vi "FL_Preprocess_and_save_incrementally_TDMS.vi"(0 "Temporary file output path":path, 1 "Loop iteration":i32, 2 "Mouse face dir. swap":bool, 3 "Loop speed in ms":u16, 4 "Save every N seconds":u32=15, 5 "error in (no error)":errorcluster, 6 "Filter type":u16(ring)=5 items=["None", "Kalman 0.50", "Kalman 0.30", "Kalman 0.12", "Savitzky-Golay 3/5", "Savitzky-Golay 3/11", "Savitzky-Golay 3/31"], 7 "Sensor read input":T3(array[cluster]), 8 "Offset":sgl, 9 "tdms file in":refnum<k34>, 10 "Pixels per mm":dbl, 11 "Data flow controls in":T2, 12 "Diagram at recording bounds":T1, 13 "Sensor board size":string="Small") -> (14 "Eff. save interval":sgl, 15 "Latest sensor output (decoded)":string[][](array[string]), 16 "Fire TTL":bool, 17 "TTL out N":u8, 18 "Current TTL status":u8, 19 "error out":errorcluster)   [LabVIEW 2016]
uses:
  <vilib>/Utility/miscctls.llb/LVBoundsTypeDef.ctl
  SW_Globals.vi
  <vilib>/Utility/file.llb/Write Delimited Spreadsheet (string).vi
panel:
  out "Bytes return count":u32
  out "VISA error out":errorcluster
  out "Output to the external terminal":string
  in  "Max chunk size":i64=100000
  in  "Number of the file chunk":u32
  out "Chunk size (in bytes)":i64
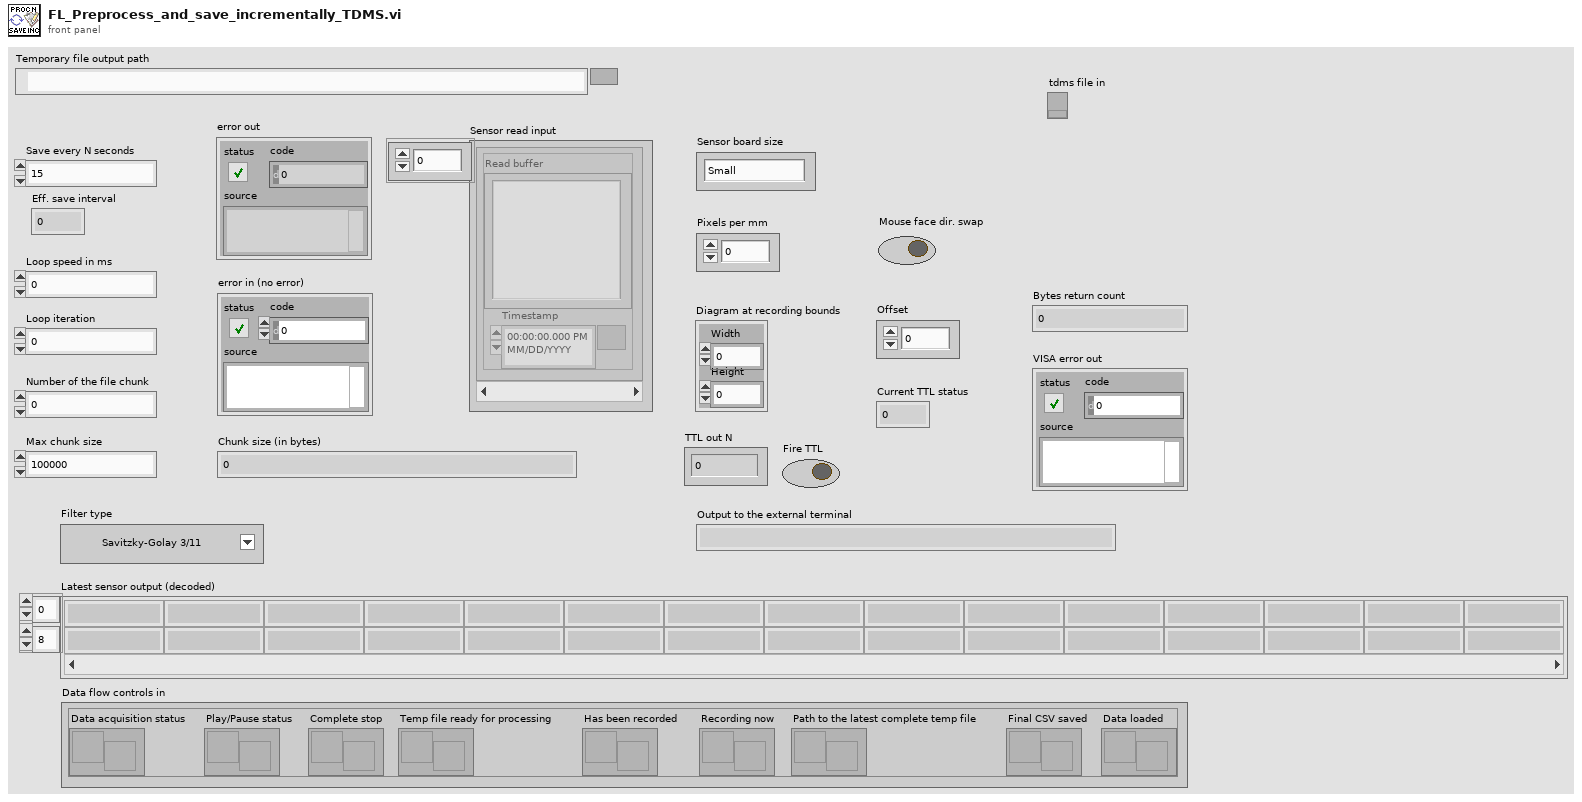
[diagram p1: front panel]
types:
  T1 = typedef "LVBoundsTypeDef.ctl" = cluster{"Width":u32, "Height":u32}
  T2 = cluster{"Data acquisition status":refnum<notifier>, "Play/Pause status":refnum<notifier>, "Complete stop":refnum<notifier>, "Temp file ready for processing":refnum<notifier>, "Has been recorded":refnum<notifier>, "Recording now":refnum<notifier>, "Path to the latest complete temp file":refnum<notifier>, "Final CSV saved":refnum<notifier>, "Data loaded":refnum<notifier>}
  T3 = cluster{"Read buffer":string, "Timestamp":timestamp}[]
  T4 = cluster{"ms since ON":u32, "delta time":u32, "X1":sgl, "Y1":sgl, "X2":sgl, "Y2":sgl, "TTL inputs":u8, "TTL outputs":u8, "Frame timestamp":timestamp, "Frame OK":bool}
  T5 = cluster{"X1 filtered":dbl, "Y1 filtered":dbl, "X2 filtered":dbl, "Y2 filtered":dbl, "X1 raw":dbl, "Y1 raw":dbl, "X2 raw":dbl, "Y2 raw":dbl}
  T6 = cluster{"R from center":dbl, "sin(a)":dbl, "Mouse Xc":dbl, "Mouse Yc":dbl, "X1-X2":dbl, "Y1-Y2":dbl, "Cage Xc":dbl, "Cage Yc":dbl}
  T7 = cluster{"R from center":dbl, "phi (mouse angular position in the cage)":dbl, "alpha (mouse rot. angle)":sgl, "X":dbl, "Y":dbl, "theta (from center towards mouse)":dbl, "beta (cage rot. against mouse)":sgl, "w (mouse angle to wall)":dbl}
  T8 = cluster{"Zone[1]":bool, "Zone[2]":bool, "Zone[3]":bool, "Zone[4]":bool, "Zone[5]":bool, "Zone[6]":bool, "Zone[7]":bool, "Zone[8]":bool, "Zone[9]":bool, "Zone[10]":bool, "Zone[11]":bool, "Zone[12]":bool, "Zone[13]":bool}
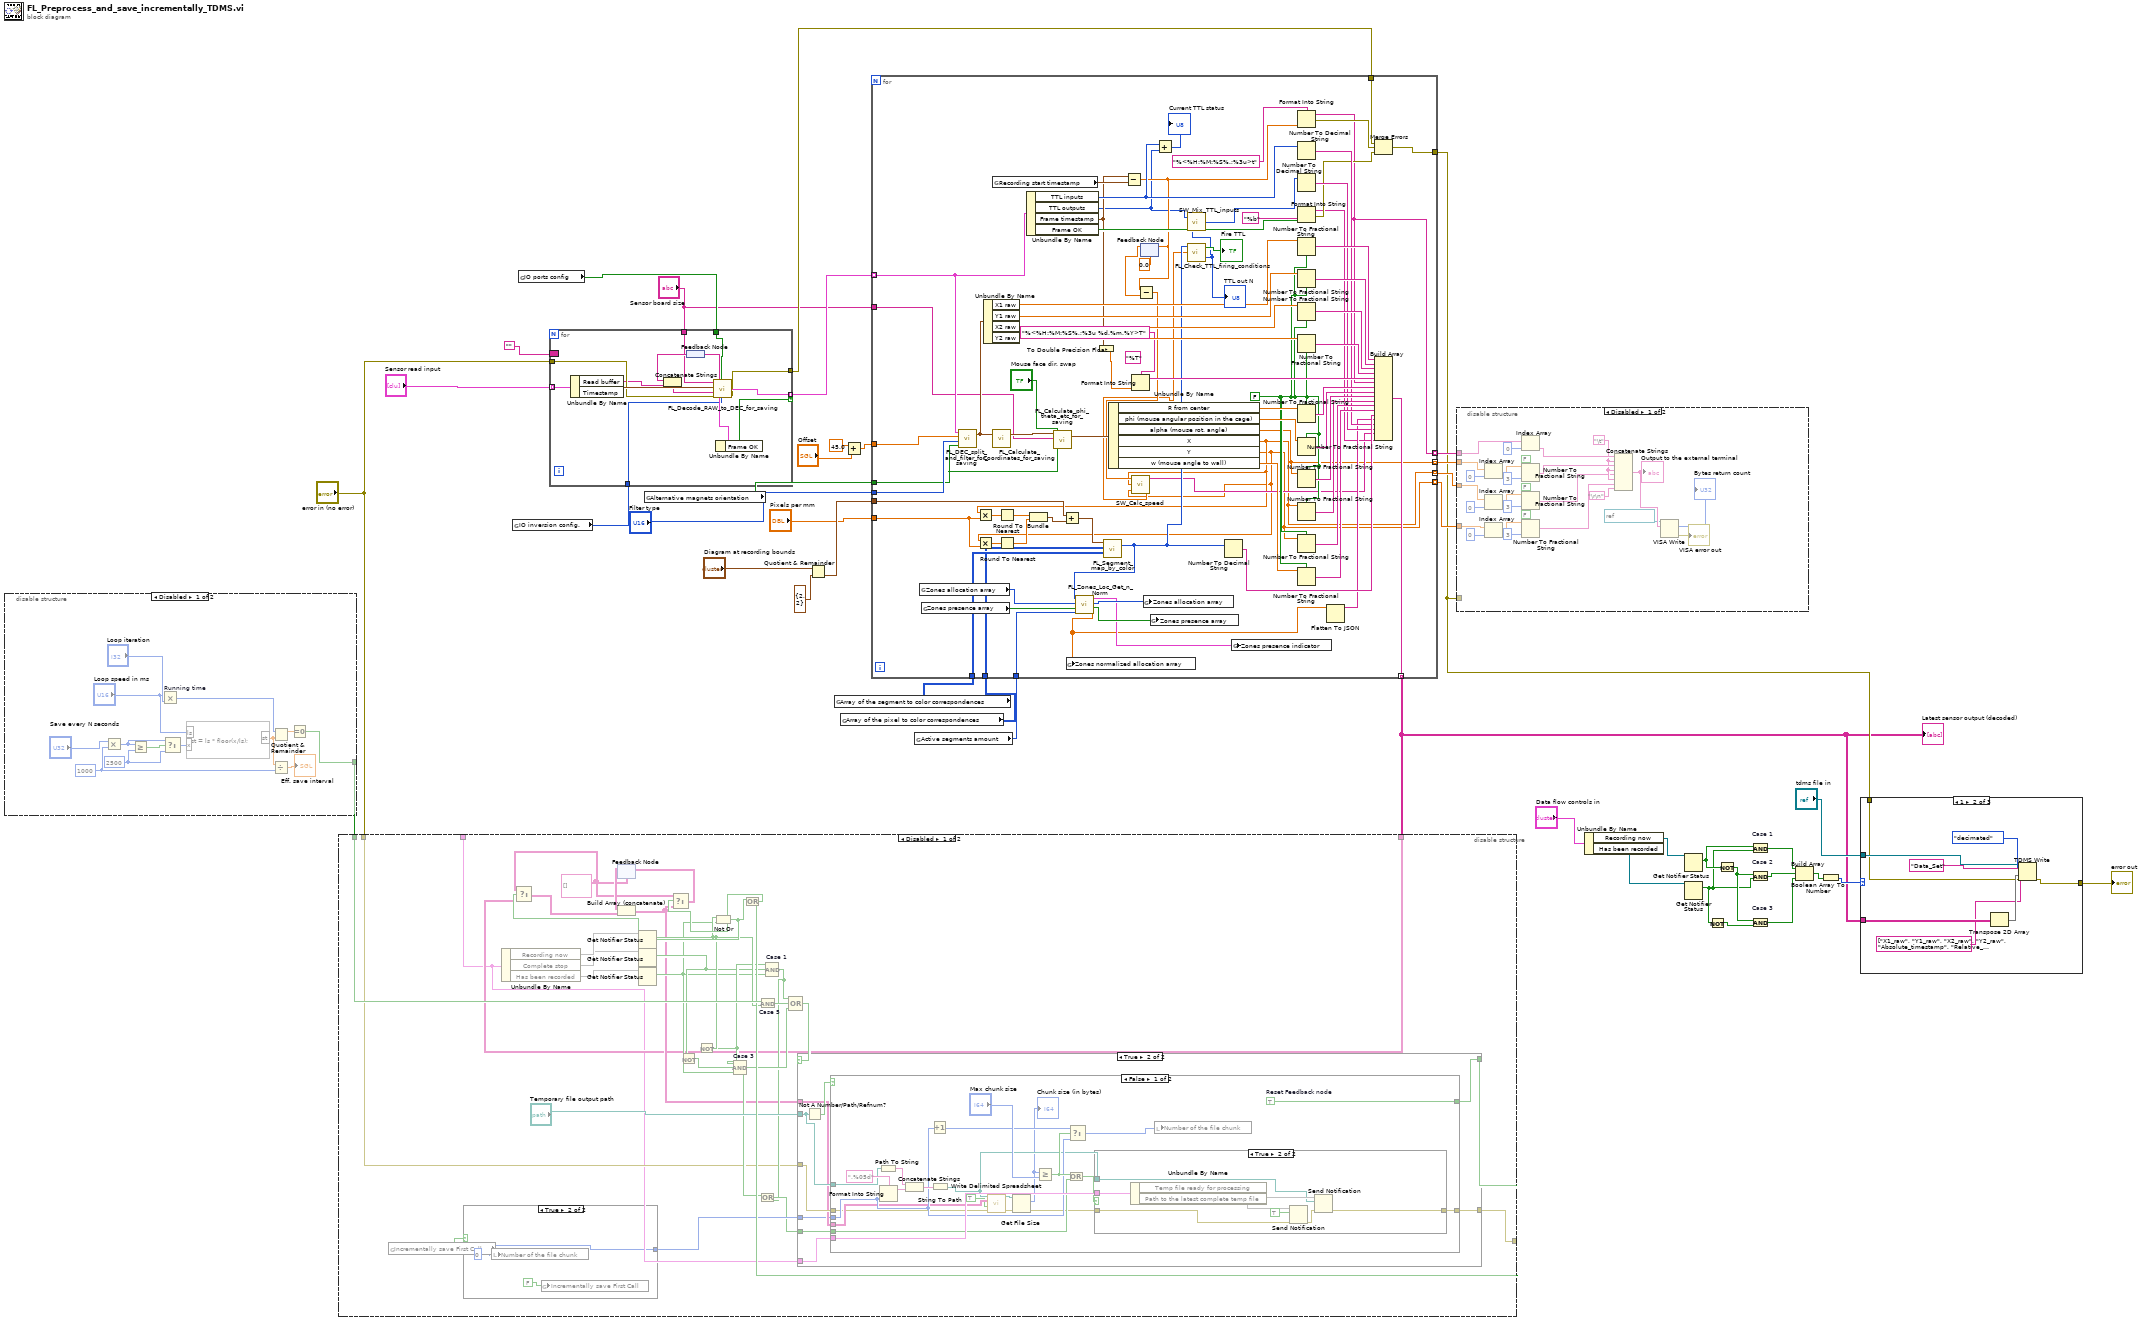
[diagram p0: block diagram]
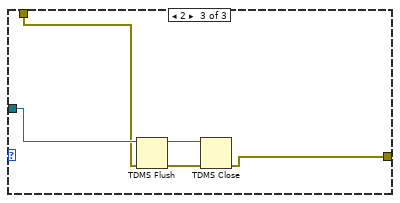
[diagram p3: hidden frame]
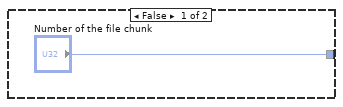
[diagram p4: hidden frame]
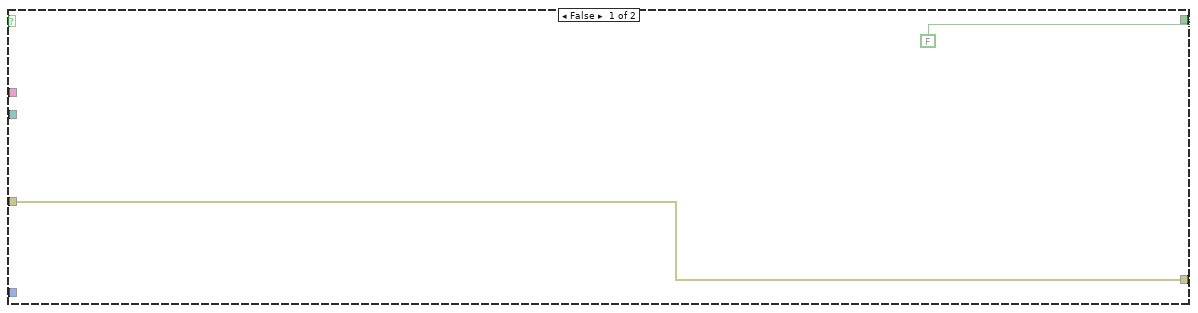
[diagram p5: hidden frame]
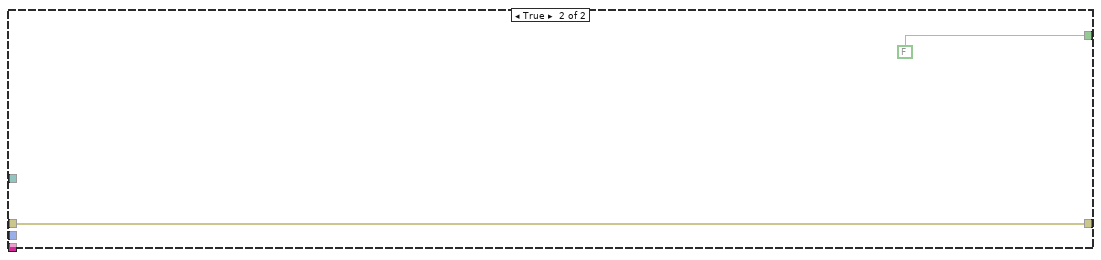
[diagram p7: hidden frame]
diagram:
  n1 = disable-structure shown="Disabled" {
    disable-tunnel: [w52 _] -> w41
    frame Disabled {
      w42 = u32 1000 ("y")
      w49 = 2500
      n2 = Multiply(x="Save every N seconds", y=w42) -> (x*y=w45:u32)
      n3 = Greater Or Equal?(x=w45, y=w49) -> (x >= y?=w50:bool)
      n4 = Multiply "Running time"(x="Loop speed in ms", y="Loop iteration") -> (x*y=w53:i32)
      n5 = Select(t=w45, s=w50, f=w49) -> (s? t:f=w47:u32)
      n6 = formula code="st = ls * floor(x/ls);"("ls"="Loop speed in ms", "x"=w47) -> ("st"=w44:dbl)
      n7 = Divide(x=w44, y=w42) -> (x/y=→"Eff. save interval":dbl)
      n8 = Quotient & Remainder(x=w53, y=w44) -> (x-y*floor(x/y)=w51:dbl)  [unwired: 1 out]
      n9 = Equal To 0?(x=w51) -> (x = 0?=w52:bool)
    }
    frame Enabled {
    }
  }
  n10 = global read "SW_Globals.vi" "IO inversion config."() -> (w21:u16)
  n11 = global read "SW_Globals.vi" "IO ports config"() -> (w24:bool[])
  n12 = for {
    tunnel: "Sensor read input" -> [w67] mode=indexing
    border: "" -> [_]
    tunnel: [w62] -> w38 mode=indexing if=w61
    tunnel: [w60] -> w39
    tunnel: "error in (no error)" -> [w59]
    tunnel: "Sensor board size" -> [w58]
    tunnel: w24 -> [w57]
    tunnel: w21 -> [w55]
    n13 = Unbundle By Name(w67) -> ("Read buffer"=w56:string, "Timestamp"=w66:timestamp)
    n14 = feedback #1() -> (w63:string)
    n15 = Concatenate Strings(w63, w56) -> (w65:string)
    n16 = call "FL_Decode_RAW_to_DEC_for_saving.vi"("Sensor board size"=w58, "IO ports config"=w57, "Input timestamp"=w66, "Input string"=w65, "IO inversion config."=w55, "Error In"=w59) -> ("Output string leftover"=w64:string, "DEC output cluster"=w62:T4, "Error Out"=w60:errorcluster)
    n17 = feedback-in #1(w64) -> ()
    n18 = Unbundle By Name(w62) -> ("Frame OK"=w61:bool)
  }
  n19 = global read "SW_Globals.vi" "Alternative magnets orientation"() -> (w23:bool)
  n20 = Quotient & Remainder(x="Diagram at recording bounds", y=T1 {"Width"=2, "Height"=2}) -> (floor(x/y)=w33:T1)  [unwired: 1 out]
  n21 = global read "SW_Globals.vi" "Array of the segment to color correspondences"() -> (w31:u32[][])
  n22 = global read "SW_Globals.vi" "Array of the pixel to color correspondences"() -> (w30:u32[][])
  n23 = Add(x=sgl 45.0, y="Offset") -> (x+y=w26:sgl)
  n24 = global read "SW_Globals.vi" "Active segments amount"() -> (w28:u8)
  n25 = for {
    tunnel: w38 -> [w144] mode=indexing
    tunnel: [w118] -> w3
    tunnel: w39 -> [w117]
    tunnel: [w72] -> w1 mode=indexing
    tunnel: "Filter type" -> [w116]
    tunnel: w33 -> [w109]
    tunnel: "Pixels per mm" -> [w115]
    tunnel: w31 -> [w107]
    tunnel: w30 -> [w106]
    tunnel: w28 -> [w102]
    tunnel: w26 -> [w93]
    tunnel: w23 -> [w78]
    tunnel: "Sensor board size" -> [w77]
    tunnel: [w71] -> w19 mode=indexing
    tunnel: [w70] -> w18 mode=indexing
    tunnel: [w69] -> w17 mode=indexing
    tunnel: [w68] -> w20 mode=indexing
    w120 = FALSE ("use system decimal point (T)")
    (unwired) "%T" ("format string")
    n26 = global read "SW_Globals.vi" "Zones allocation array"() -> (w103:i32[])
    n27 = global read "SW_Globals.vi" "Zones presence array"() -> (w101:bool[])
    n28 = call "FL_DEC_split_and_filter_for_saving.vi"("Alternative magnets orientation"=w78, "Filter type"=w116, "Offset"=w93, "DEC input cluster"=w144) -> ("Magnets coords"=w146:T5)  [unwired: 1 in]
    n29 = Unbundle By Name(w146) -> ("X1 raw"=w137:dbl, "Y1 raw"=w135:dbl, "X2 raw"=w133:dbl, "Y2 raw"=w130:dbl)
    n30 = call "FL_Calculate_Coordinates_for_saving.vi"("Magnets coords in"=w146) -> ("Output cluster of data"=w145:T6)  [unwired: 2 in]
    n31 = global read "SW_Globals.vi" "Recording start timestamp"() -> (w143:timestamp)
    n32 = Unbundle By Name(w144) -> ("TTL inputs"=w89:u8, "TTL outputs"=w74:u8, "Frame timestamp"=w81:timestamp, "Frame OK"=w141:bool)
    n33 = call "FL_Calculate_phi_theta_etc_for_saving.vi"("Use alternative magnets orientation"=w78, "Mouse face dir. swap"="Mouse face dir. swap", "Sensor board size"=w77, "Input cluster of data"=w145) -> ("Output data cluster"=w138:T7)  [unwired: 1 in]
    n34 = To Double Precision Float(number=w81) -> (double precision float=w80:dbl)
    n35 = Unbundle By Name(w138) -> ("R from center"=w129:dbl, "phi (mouse angular position in the cage)"=w127:dbl, "alpha (mouse rot. angle)"=w71:sgl, "X"=w70:dbl, "Y"=w69:dbl, "w (mouse angle to wall)"=w122:dbl)
    n36 = Multiply(x=w70, y=w115) -> (x*y=w114:dbl)
    n37 = Multiply(x=w69, y=w115) -> (x*y=w113:dbl)
    n38 = Round To Nearest(number=w114) -> (nearest integer value=w112:dbl)
    n39 = Round To Nearest(number=w113) -> (nearest integer value=w111:dbl)
    n40 = Bundle(w112, w111) -> (w110:cluster{dbl, dbl})  [unwired: 1 in]
    n41 = Add(x=w109, y=w110) -> (x+y=w108:cluster{dbl, dbl})
    n42 = call "FL_Segment_map_by_color.vi"("Array of the segment to color correspondences"=w107, "Array of the pixel to color correspondences"=w106, "Mouse abs. coordinates, pix"=w108) -> ("Current segment' number"=w91:u32)  [unwired: 1 in, 1 out]
    n43 = call "FL_Zones_Loc_Get_n_Norm.vi"("Amount of active segments"=w102, "Zones presence array in"=w101, "Zones allocation array in"=w103, "Current segment' number"=w91) -> ("Zones normalized allocation array out"=w94:dbl[], "Zones presence array out"=w99:bool[], "Zones allocation array out"=w100:i32[], "Zones presence indicator cluster out"=w98:T8)  [unwired: 4 in]
    n44 = global write "SW_Globals.vi" "Zones normalized allocation array"(w94) -> ()
    n45 = Subtract(x=w81, y=w143) -> (x-y=w85:dbl)
    n46 = Format Into String(format string="%<%H:%M:%S%,;%3u %d.%m.%Y>T", w80) -> (resulting string=w139:string)  [unwired: 2 in, 1 out]
    n47 = feedback-in #2(w85) -> ()
    n48 = feedback #2(0.0) -> (w86:dbl)
    n49 = Subtract(x=w85, y=w86) -> (x-y=w83:dbl)
    n50 = call "SW_Calc_speed.vi"("Y coord, mm"=w69, "X coord, mm"=w70, "Time per frame, s"=w83) -> ("Mouse speed for TTL detection, mm/s"=w76:dbl, "Mouse speed for saving, mm/s"=w82:string)  [unwired: 1 out]
    n51 = global write "SW_Globals.vi" "Zones allocation array"(w100) -> ()
    n52 = global write "SW_Globals.vi" "Zones presence array"(w99) -> ()
    n53 = Add(x=w89, y=w74) -> (x+y=→"Current TTL status":u8)
    n54 = call "FL_Check_TTL_firing_conditions.vi"("Current speed, mm/s"=w76, "Current segment' number (last value)"=w91) -> ("TTL out N"=w73:u8, "Fire TTL"=→"Fire TTL":bool)  [unwired: 1 in]
    "TTL out N" <- w73
    n55 = call "SW_Mix_TTL_inputs.vi"("TTL input 2"=w73, "TTL input 1"=w74) -> ("TTL mixed output"=w75:u8)
    n56 = Number To Decimal String(number=w91) -> (decimal integer string=w105:string)  [unwired: 1 in]
    n57 = global write "SW_Globals.vi" "Zones presence indicator"(w98) -> ()
    n58 = Format Into String(format string="%<%H:%M:%S%.;%3u>t", w85) -> (resulting string=w68:string, error out=w119:errorcluster)  [unwired: 2 in]
    n59 = Number To Decimal String(number=w89) -> (decimal integer string=w96:string)  [unwired: 1 in]
    n60 = Number To Decimal String(number=w75) -> (decimal integer string=w97:string)  [unwired: 1 in]
    n61 = Format Into String(format string="%b", w141) -> (resulting string=w84:string, error out=w92:errorcluster)  [unwired: 2 in]
    n62 = Number To Fractional String(use system decimal point (T)=w120, number=w137) -> (F-format string=w136:string)  [unwired: 2 in]
    n63 = Number To Fractional String(use system decimal point (T)=w120, number=w135) -> (F-format string=w134:string)  [unwired: 2 in]
    n64 = Number To Fractional String(use system decimal point (T)=w120, number=w133) -> (F-format string=w132:string)  [unwired: 2 in]
    n65 = Number To Fractional String(use system decimal point (T)=w120, number=w130) -> (F-format string=w131:string)  [unwired: 2 in]
    n66 = Number To Fractional String(use system decimal point (T)=w120, number=w129) -> (F-format string=w128:string)  [unwired: 2 in]
    n67 = Number To Fractional String(use system decimal point (T)=w120, number=w127) -> (F-format string=w126:string)  [unwired: 2 in]
    n68 = Number To Fractional String(use system decimal point (T)=w120, number=w71) -> (F-format string=w125:string)  [unwired: 2 in]
    n69 = Number To Fractional String(use system decimal point (T)=w120, number=w70) -> (F-format string=w124:string)  [unwired: 2 in]
    n70 = Number To Fractional String(use system decimal point (T)=w120, number=w69) -> (F-format string=w123:string)  [unwired: 2 in]
    n71 = Number To Fractional String(use system decimal point (T)=w120, number=w122) -> (F-format string=w121:string)  [unwired: 2 in]
    n72 = Flatten To JSON(anything=w94) -> (JSON string=w95:string)  [unwired: 2 in, 1 out]
    n73 = Merge Errors(w117, w119, w92) -> (w118:errorcluster)
    n74 = Build Array(w136, w134, w132, w131, w139, w68, w128, w126, w125, w124, w123, w121, w105, w95, w96, w97, w82, w84) -> (w72:string[])
  }
  "Latest sensor output (decoded)" <- w1
  n75 = disable-structure shown="Disabled" {
    disable-tunnel: w41 -> [w174 _]
    disable-tunnel: "error in (no error)" -> [w151 _]
    disable-tunnel: [w150 _] -> _
    disable-tunnel: w1 -> [w148 _]
    disable-tunnel: _ -> [w147 _]
    frame Disabled {
      w162 = string[][] []
      n76 = global read "SW_Globals.vi" "Incrementally save First Call"() -> (w149:bool)
      n77 = case shown="True" w149 {
        tunnel: ["Number of the file chunk" w178] -> w165
        frame False {
        }
        frame True {
          w178 = 0 ("Number of the file chunk")
          n78 = local write "Number of the file chunk"(w178) -> ()
          n79 = global write "SW_Globals.vi" "Incrementally save First Call"(FALSE ("Incrementally save First Call")) -> ()
        }
      }
      n80 = Unbundle By Name(w147) -> ("Recording now"=w169, "Complete stop"=w168, "Has been recorded"=w167)
      n81 = feedback #3(w162) -> (w172:string[][])
      n82 = Get Notifier Status(notifier=w169) -> (current notification=w159:bool)  [unwired: 1 in, 4 out]
      n83 = Get Notifier Status(notifier=w168) -> (current notification=w157:bool)  [unwired: 1 in, 4 out]
      n84 = Get Notifier Status(notifier=w167) -> (current notification=w156:bool)  [unwired: 1 in, 4 out]
      n85 = Not(x=w157) -> (.not. x?=w155:bool)
      n86 = Not(x=w159) -> (.not. x?=w158:bool)
      n87 = Not Or(1:w156, 2:w159) -> (0:w161:bool)
      n88 = Select(t=w162, s=w161, f=w148) -> (s? t:f=w163:string[][])
      n89 = Build Array (concatenate)(w172, w163) -> (w152:string[][])
      n90 = Compound Arithmetic op=AND "Case 3"(w158, w155, w156) -> (w164:bool)
      n91 = And "Case 5"(x=w174, y=w159) -> (x .and. y?=w175:bool)
      n92 = Compound Arithmetic op=AND "Case 1"(w158, w157, w156) -> (w153:bool)
      n93 = Or(x=w164, y=w153) -> (x .or. y?=w154:bool)
      n94 = Compound Arithmetic op=OR(w153, w175, w164) -> (w173:bool)
      n95 = case shown="True" w173 {
        tunnel: "Temporary file output path" -> [_ w188]
        tunnel: [FALSE w187] -> w170
        tunnel: w151 -> [w179 w186]
        tunnel: [w179 w185] -> w150
        tunnel: w152 -> [_ w184]
        tunnel: w147 -> [_ w183]
        tunnel: w165 -> [_ w182]
        tunnel: w154 -> [_ w181]
        frame False {
        }
        frame True {
          n96 = Not A Number/Path/Refnum?(number/path/refnum=w188) -> (NaN/Path/Refnum?=w189:bool)
          n97 = case shown="False" w189 {
            tunnel: w188 -> [w204 _]
            tunnel: [w195 FALSE] -> w187
            tunnel: w186 -> [w191 w222]
            tunnel: [w202 w222] -> w185
            tunnel: w184 -> [w197 _]
            tunnel: w182 -> [w199 _]
            tunnel: w183 -> [w209 _]
            tunnel: w181 -> [w200 _]
            frame False {
              w195 = TRUE  # Reset Feedback node
              n98 = Path To String(path=w204) -> (string=w206:string)
              n99 = Format Into String(format string=".%05d", w199) -> (resulting string=w207:string)  [unwired: 2 in, 1 out]
              n100 = Concatenate Strings(w206, w207) -> (w208:string)
              n101 = Increment(x=w199) -> (x+1=w211:u32)
              n102 = String To Path(string=w208) -> (path=w198:path)
              n103 = call-poly <vilib>:"Write Delimited Spreadsheet.vi"("file path (dialog if empty)"=w198, "2D data"=w197, "append to file? (new file:F)"=TRUE, "error in (no error)"=w191) -> ("new file path (Not A Path if cancelled)"=w194:path, "error out"=w193:errorcluster)  [unwired: 10 in]
              n104 = Get File Size(file=w194, error in=w193) -> (size (in bytes)=w190:i64, 0:w192:errorcluster)  [unwired: 1 out]
              "Chunk size (in bytes)" <- w190
              n105 = Greater Or Equal?(x=w190, y="Max chunk size") -> (x >= y?=w203:bool)
              n106 = Or(x=w203, y=w200) -> (x .or. y?=w201:bool)
              n107 = Select(t=w211, s=w203, f=w199) -> (s? t:f=w210:u32)
              n108 = case shown="True" w201 {
                tunnel: w209 -> [_ w221]
                tunnel: w198 -> [_ w215]
                tunnel: w192 -> [w213 w217]
                tunnel: [w213 w216] -> w202
                frame False {
                }
                frame True {
                  n109 = Unbundle By Name(w221) -> ("Temp file ready for processing"=w220, "Path to the latest complete temp file"=w219)
                  n110 = Send Notification(notification=TRUE, notifier=w220, error in (no error)=w217) -> (error out=w218:errorcluster)  [unwired: 1 out]
                  n111 = Send Notification(notification=w215, notifier=w219, error in (no error)=w218) -> (error out=w216:errorcluster)  [unwired: 1 out]
                }
              }
              n112 = local write "Number of the file chunk"(w210) -> ()
            }
            frame True {
            }
          }
        }
      }
      n113 = Or(x=w161, y=w170) -> (x .or. y?=w160:bool)
      n114 = Select(t=w162, s=w160, f=w152) -> (s? t:f=w171:string[][])
      n115 = feedback-in #3(w171) -> ()
    }
    frame Enabled {
    }
  }
  n116 = disable-structure shown="Disabled" {
    disable-tunnel: w20 -> [w250 _]
    disable-tunnel: w19 -> [w245 _]
    disable-tunnel: w18 -> [w244 _]
    disable-tunnel: w17 -> [w243 _]
    disable-tunnel: w3 -> [_ _]
    frame Disabled {
      w231 = "\t"
      n117 = Index Array(array=w245, index=0) -> (element=w242:sgl)
      n118 = Index Array(array=w244, index=0) -> (element=w237:dbl)
      n119 = Index Array(array=w243, index=0) -> (element=w234:dbl)
      n120 = Index Array(array=w250, index=0) -> (element=w233:string)
      n121 = Number To Fractional String(use system decimal point (T)=FALSE, number=w242, precision (6)=i16 3) -> (F-format string=w232:string)  [unwired: 1 in]
      n122 = Number To Fractional String(use system decimal point (T)=FALSE, number=w237, precision (6)=i16 3) -> (F-format string=w230:string)  [unwired: 1 in]
      n123 = Number To Fractional String(use system decimal point (T)=FALSE, number=w234, precision (6)=i16 3) -> (F-format string=w229:string)  [unwired: 1 in]
      n124 = Concatenate Strings(w233, w231, w232, w231, w230, w231, w229, "\r\n") -> (w227:string)
      "Output to the external terminal" <- w227
      n125 = VISA Write(VISA resource name=refnum<visa-resource-name> "COMTEST", write buffer=w227) -> (return count=→"Bytes return count":u32, error out=→"VISA error out":errorcluster)  [unwired: 1 in, 1 out]
    }
    frame Enabled {
    }
  }
  n126 = Unbundle By Name("Data flow controls in") -> ("Recording now"=w15:refnum<notifier>, "Has been recorded"=w14:refnum<notifier>)
  n127 = Get Notifier Status(notifier=w15) -> (current notification=w13:bool)  [unwired: 1 in, 4 out]
  n128 = Get Notifier Status(notifier=w14) -> (current notification=w10:bool)  [unwired: 1 in, 4 out]
  n129 = Not(x=w10) -> (.not. x?=w11:bool)
  n130 = Not(x=w13) -> (.not. x?=w12:bool)
  n131 = And "Case 1"(x=w13, y=w10) -> (x .and. y?=w9:bool)
  n132 = And "Case 2"(x=w12, y=w10) -> (x .and. y?=w8:bool)
  n133 = And "Case 3"(x=w12, y=w11) -> (x .and. y?=w7:bool)
  n134 = Build Array(w9, w8, w7) -> (w5:bool[])
  n135 = Boolean Array To Number(Boolean array=w5) -> (number=w6:u32)
  n136 = case shown="1" w6 {
    tunnel: "tdms file in" -> [_ w256 w264]
    tunnel: w3 -> [w251 w255 w261]
    tunnel: [w251 w254 w260] -> w2
    tunnel: w1 -> [_ w253 _]
    frame 4, Default {
    }
    frame 1 {
      n137 = Transpose 2D Array(2D array=w253) -> (transposed array=w257:string[][])
      n138 = TDMS Write(0:w256, 1:enum16{"decimated", "interleaved"}."decimated" ("data layout (0:decimated)"), 5:"Data_Set" ("group name in (Untitled)"), 7:string[] ["X1_raw", "Y1_raw", "X2_raw", "Y2_raw", "Absolute_timestamp", "Relative_timestamp", "R", "phi", "alpha", "X", "Y", "w", "Current_zone", "Zones_preference", "TTL_inputs", "TTL_outputs", "Speed_mm_per_s", "Frame_OK"] ("Columns Names"), 9:w257, 11:w255) -> (15:w254:errorcluster)  [unwired: 3 out]
    }
    frame 2 {
      n139 = TDMS Flush(4:w261, 7:w264) -> (0:w262:errorcluster, 3:w263:refnum<k34>)
      n140 = TDMS Close(8:w262, 11:w263) -> (0:w260:errorcluster)  [unwired: 1 out]
    }
  }
  "error out" <- w2
